vi "写入database.vi"(8 "error in (no error)":errorcluster, 11 "data":T1) -> (0 "error out":errorcluster)   [LabVIEW 2022 SP3, in "LS-H600-TCP Client.lvlib" / "LS-H600-TCP Client.lvclass"]
uses:
  LS-H600-TCP Client.lvclass
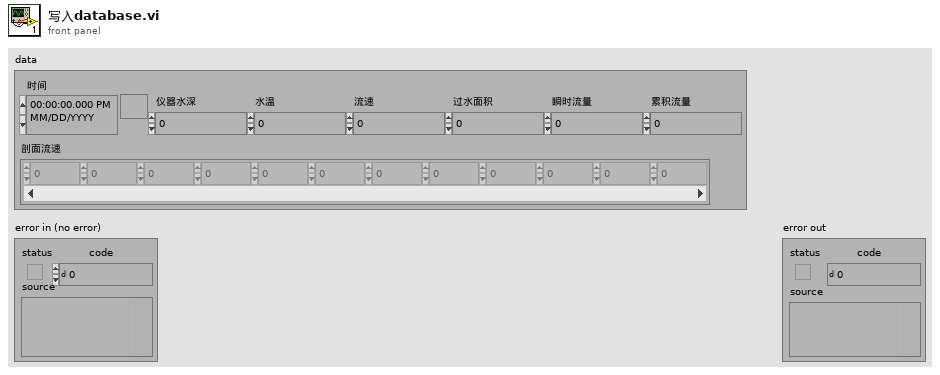
[diagram p1: front panel]
types:
  T1 = cluster{"时间":timestamp, "仪器水深":dbl, "水温":dbl, "流速":dbl, "过水面积":dbl, "瞬时流量":dbl, "累积流量":dbl, "剖面流速":dbl[]}
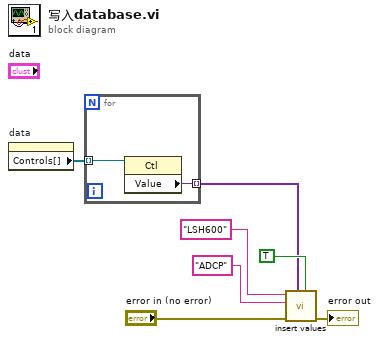
[diagram p0: block diagram]
diagram:
  n1 = property on="data" class="Clust (strict)"() -> ("Controls[]"=w5:refnum<vi>[])  [unwired: 2 in, 2 out]
  n2 = for {
    tunnel: w5 -> [w9] mode=indexing
    tunnel: [w8] -> w4 mode=indexing
    n3 = property class="Ctl"(reference=w9) -> ("Value"=w8:variant)  [unwired: 1 in, 2 out]
  }
  n4 = call "insert values.vi"("是否创建唯一键"=TRUE, "data"=w4, "错误输入（无错误）"="error in (no error)", "database"="ADCP", "Tabe Name"="LSH600") -> ("错误输出"=→"error out":errorcluster)  [unwired: 6 in]
